vi "CRYReplace Curve Name of Steps.vi"(7 "Option flg":bool, 8 "Steps In":T1[](array[typedef]) {"Repeat State Array"."Start" format="%#_5g"; "Y dB ref" format="%.1f"; "Y data" items=["dB", "Lin"]; "Start" format="%#_5g"}, 9 "Step Category":string, 10 "New Name":string[](array[string]), 11 "Old Name":string[](array[string])) -> (3 "Steps Out":T1[](array[typedef]) {"Repeat State Array"."Start" format="%#_5g"; "Y dB ref" format="%.1f"; "Y data" items=["dB", "Lin"]; "Start" format="%#_5g"})   [LabVIEW 2013]
uses:
  Typedef Control/CRYStep.ctl
  CRYProject/CRYProject Editor Global.vi
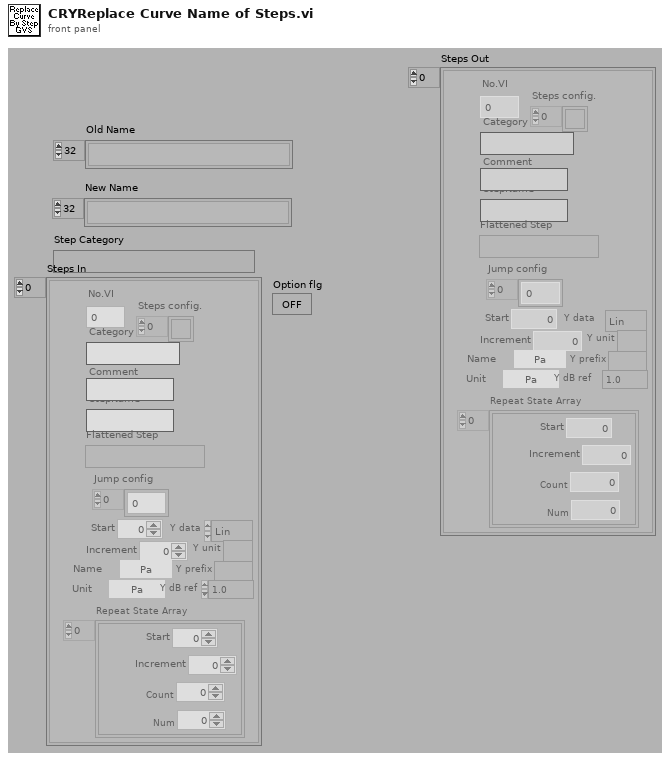
[diagram p1: front panel]
types:
  T1 = typedef "CRYStep.ctl" = cluster{"No.VI":i32, "Category":string, "StepName":string, "Seq setup flattened":string, "Comment":string, "Steps config.":bool[], "Jump config":i32[], "Start":dbl, "Increment":dbl, "Name":string, "Unit":string, "Y data":u16, "Y prefix":string, "Y dB ref":dbl, "Y unit":string, "Repeat State Array":cluster{"Start":dbl, "Increment":dbl, "Count":i32, "Num":i32}[]}
  T2 = typedef "CRYAcquisition Cluster.ctl" = cluster{"Mode":u16, "Name":string, "use ch name":bool, "Record Time":dbl, "hide rec":bool, "hide play":bool, "rec delay":dbl, "rec pad":dbl, "dcc units":i8, "sine gen setting":string, "scope_fft setting":string, "voltmeter setting":string, "rta setting":string, "trig offset(sec)":dbl, "triggered  record":bool, "trig level":dbl, "trig unit":u8, "trig slop":bool, "trig timeout(sec)":dbl, "add record":bool, "EQ":bool, "record table":string[][], "play table":string[][], "trig channel":string, "Help":string}
  T3 = typedef "CRYAnalysis Cluster.ctl" = cluster{"Name":string, "Harmonics":dbl[], " Algorithm":u16, "delay":dbl, "THD(%)":bool, "Rub&Buzz":bool, "Imp":bool, "Imp Ref resistor":dbl, "Y data":u16, "Y prefix":string, "Y unit":string, "Y dB ref":dbl, "Custom Curve Names":string[], "har list items":string[], "Envelope":bool, "use custom unit":bool, "autodelay ch":dbl, "impulse":bool, " start ms":dbl, " stop ms":dbl, "Scaling":i32, "Default Overlap ":bool, "Advanced View":bool, "Loose Particle":bool, "Use default":bool, "Auto-Correlation(Stimulus)":bool, "Auto-Correlation(Response)":bool, "Deconvolved Response":bool, "Mic Current":bool, "M List Vaiues":u16, "Type":u16, "Delay Method":u16, "Apply Correction Out":bool, "Apply Correction In":bool, "Harmonics @ meas.frq":bool, "THD Normalized(%)":bool, "Total Distortion":bool, "THD+Noise(%)":bool, "Rub&Buzz Norm'd(%)":bool, "Standard Error":bool, "Confidence Limits":bool, "Total Diff":bool, "Total Noise":bool, "Total DFD(%)":bool, "Total IMD(%)":bool, "Total IM":bool, "Total DFD+Noise(%)":bool, "Use Channel Name":bool, "Waveform In":string, "Waveform Out":string, "Method":u16, "Spectral Scaling":u16, "Appliied Unit":u16, "Length Unit":u16, "Applied Units":u16, "Sens Item":u16, "Tab":i32, "Distance Unit":u16, "discard cycles":dbl, "Weigting":string, "Averaging Time":dbl, "Max duration":dbl, "Min duration":dbl, "Attack Threshold":dbl, "Hysteresis Up":dbl, "Fmin(Hz)":dbl, "Fmax(Hz)":dbl, "Freq.Resolution":dbl, "Over-samples Res.":dbl, "Win Resolution":dbl, "distance":dbl, "samples":dbl, "Overlap":dbl, "Record Length":dbl, "No.of FFTs":dbl, "Hz":dbl, "record delay":dbl, " Std Err":dbl, "Response":bool, "Coherent Power*":bool, "Stimulus":bool, "Measurement Confidence":bool, "Auto Spectrum(Response)*":bool, "Auto Spectrum(Stimulus)*":bool, "Cross Spectrum*":bool, "functions":bool, "Frequency Response":bool, "Non-Coherent Power*":bool, "Coherence (%)":bool, "Non-Coherence (%)":bool, "Signal-Noise Ratio (dB)":bool, "Non-Coherenct Distirtion*":bool, "Result Waveforms":bool, "Coupling":bool, "Averaging":u16, "Harmonics":i32, "Custom Curve Names":i32, "unLabel":string, "Custom Curve Names":string, "Unit":string, "Total IMD + Noise(%) ":bool, "ResponseMe":u16, "Intermod":dbl[], "Diff\n":dbl[], "Cross-Correlation":bool, "IM list items":string[], "Diff list items":string[], "TSR Window Type":string, "Help":string, "Custom Curve IDs":i32[], "Default Curve Names":string[], "Loose Particle waveform":bool, "Perceptual Rub&Buzz":bool, "Imp Auto Mode":u16, "Mic Auto Mode":u16, "Mic Ref resistor":dbl, "Curve Resolution":u16, "Curve Resolution Hz":dbl, "Polarity":bool}
  T4 = typedef "CRYStimulus Cluster.ctl" = cluster{"StimulusType":string, "UseMLValArray":u16[], "ML_axisArray":u16[], "MLValLevelNameArray":string[], "Level(U)Array":dbl[], "Start(Stop)FreqArray":dbl[], "Start(Stop)AmpArray":dbl[], "StepResolutionArray":u16[], "Unit_Array":u16[], "DegValArray":dbl[], "DegUnitArray":string[], "Steps1":i32, "Cycle/step1(#)":u32, "Time/step1(s)":dbl, "Transition1":dbl, "SweepRate2":dbl, "Freq3(Hz)":dbl, "Steps3(#)":dbl, "Cycles3(#)":u32, "StepSize3":dbl, "wave time":string, "RMS_Value4":dbl, "Peak_Value4":dbl, "WavePath4":string, "RMS_unit4":string, "Peak_unit4":string, "wave Info":string, "dc_ctrl5_1":u16, "dc_ctrl5_2":u16, "dc_polar5":u16, "Max.Current":u16, "Steps5(#)":u32, "Time/Step5":dbl, "Level5":dbl, "StepsSize5Val":dbl, "StepSize5Unit":string, "SweepType":u16, "Fixed/Ratio6":u16, "Transition6":dbl, "Steps6(#)":dbl, "Cycle/Steps6(#)":u32, "Time/Steps6(s)":dbl, "Freq6(Hz)":dbl, "Difference6(Hz)":dbl, "Ratio6":string, "NoiseType7":u16, "Duration7(s)":dbl, "MinFreq7(Hz)":dbl, "MaxFreq7(Hz)":dbl, "MinFreq8(Hz)":dbl, "MaxFreq8(Hz)":dbl, "FreqRounding8":bool, "Duration8(s)":dbl, "Tones8":dbl, "RoundingVal8":dbl, "ApplyEQ":bool, "Duration(s)":dbl, "CustomStimulusName ":string, "Flatten Element Array":string[], "sine waves":cluster{"freq":dbl, "ampl":dbl, "cycles":dbl}[], "Channel Out":i32, "RatioVal6":dbl, "TabCtrl6":enum32{"Master Tone", "Slave Tone"}, "Signal Type Name":string, "Help":string, "Channel Sel":u16, "V on DUT":bool, "Output Imp":dbl, "Nominal Imp":dbl}
  T5 = typedef "CRYLimits.ctl" = cluster{"Name":string, "Tolerance":u16, "X Axis":u16, "Limits":u16, "Upper Limit":cluster{dbl, dbl}[], "Align Ref":cluster{dbl, dbl}, "Lower Limit":cluster{dbl, dbl}[], "Y data":u16, "Y unit":string, "Y dB ref":dbl, "Curve Names":string[], "Y-Resolution":u8, "Type":u16, "x float":bool, "X min-max-step":cluster{"Limit X Offset Min":dbl, "Limit X Offset Max":dbl, "Limit X Offset Step Size":dbl}, "magn/phase":u16, "Upper Limit Type":u16, "Lower Limit Type":u16, "Lim Curve axis up":u16, "Lim Curve axis lo":u16, "Data Selection Upper":u16, "Data Selection Lower":u16, "X-Resolution":u8, "Output failed point curves?":bool, "X data":u16, "X unit":string, "X dB ref":dbl, "X-Y Graph Set-up":string, "Tab Value":enum32{"Data", "Parameters"}, "Help":string, "X Up Val":dbl, "Y Up Val":dbl, "X Low Val":dbl, "Y Low Val":dbl, "Up Limit Val":dbl, "Low Limit Val":dbl, "bAdd DataName":bool, "Custom Name":string}
  T6 = typedef "CRYStatistic cluster.ctl" = cluster{"Mode":u16, "No.Ranked(BF)":i32, "No.Ranked(WF)":i32, "Absolute Margin Standard Deviation":bool, "+/- sigma Res":i32, "Margin Standard Deviation":bool, "Margin Mean":bool, "Overall Yield":bool, "Individual Limits Yield":bool, "LSL Unit":string, "USL Unit\n":string, "LSL":dbl, "USL":dbl, "Worst Fit to Average":bool, "Best Fit to Average":bool, "Ppk":bool, "Pp":bool, "Absolute Standard Deviation":bool, "+/- sigma Dat":i32, "Standard Deviation ":bool, "Mean":bool, "Min ":bool, "Max ":bool, "No.of Curves Selected":i32, "Curves":string[], " Results":string[], "Name":string, "Help":string, "Tab Value":enum32{"Setting", "Help"}, "Work in":u16, "Mode xyz":u16}
  T7 = typedef "CRYPost Processing Cluster.ctl" = cluster{"Name":string, "Op Type":u16, "Curve A":string, "Curve B":string, "Axis Mode":u16, "Work Mode":u16, "Width":u16, "Weighting win":u16, "Search Mode":u16, "Freq Mode":u16, "New Sampling Rate":dbl, "Use Default Name":bool, "x":bool, "y":bool, "z":bool, "All points":bool, "A_single val axis":u16, "B_single val axis":u16, "Use Default Value":bool, "Result Name":string, "Smoothing Width":i32, "Window":u16, "Para_dB":sgl, "Para_%":sgl, "Exponent":sgl, "Hz":dbl, "Direct Weighting":bool, "Auto Inc":bool, "Inc(deg)":i32, "Total Rotation":i32, "Ref Freq Mode":u16, "Ref Waveform":string, "Sampling Rate":dbl, "Weighting Curve":string, "Ref Freq":dbl, "Curve Group":string[], "Search Items":string[], "Custom unit info":cluster{"use custom":bool, "lin/log":u16, "unit":string, "dB ref":dbl, "common dB":u16}, "Unit":string, "Type A":enum16{"Curves", "Values", "Results", "WFM"}, "Type B":enum16{"Curves", "Values", "Results", "WFM"}, "Unary Operator":u16, "Binary Operator":u16, "Statistical Operator":u16, "Constant ":dbl, "New Resolution":u16, "user equation cluster":T8, "Help":string, "Tab Value":enum32{"Setting", "Help"}, "Zwciker_X-axis":u16, "Zwicker_spectrum":bool, "Freq Sampling Mode":u16, "Freq Sampling Rate":dbl, "Smoothing":bool, "Work in Statics":u16, "Result Data":string[]}
  T8 = typedef "CRYUser Equation Cluster.ctl" = cluster{"Custom unit input array":cluster{"use custom":bool, "lin/log":u16, "unit":string, "dB ref":dbl, "common dB":u16}[], "Custom unit results array ":cluster{"use custom":bool, "lin/log":u16, "unit":string, "dB ref":dbl, "common dB":u16}[], "Desired Result Variables":string[], "Desired Result Names":string[], "Input Curve Names":string[], "Input Curve Variables":string[], "equation":string, "Input axis":u16[], "Results axis":u16[], "# input curves":i32, "# Desired result curves ":i32, "Input Values":string[], "Result Values":string[]}
  T9 = typedef "CRYTS.ctl" = cluster{"No.TS":u16, "TS File Path":path, "TS Name":string, "EditStepName":string, "Steps":T1[], "New State":bool, "Change State":bool, "Flattened CurveLib Data":string, "Document Data":string, "EditStepNo":u16, "Operator Start File":string, "Sequence Type":string, "Sequence Language":string}
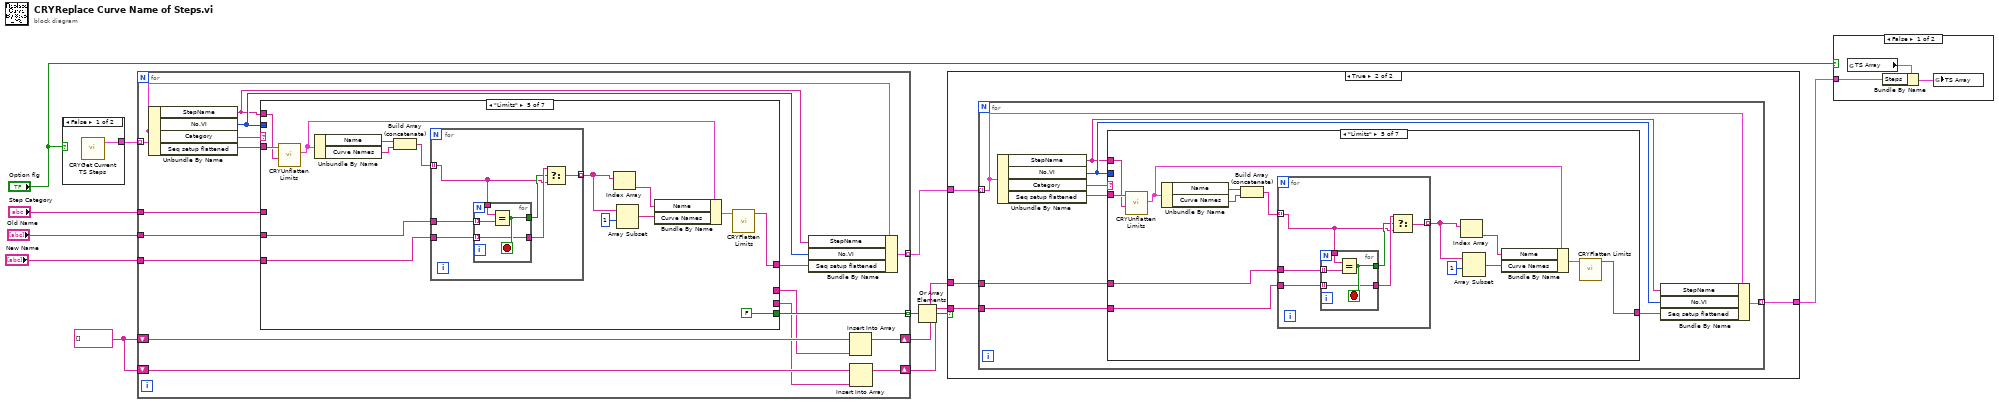
[diagram p0: block diagram]
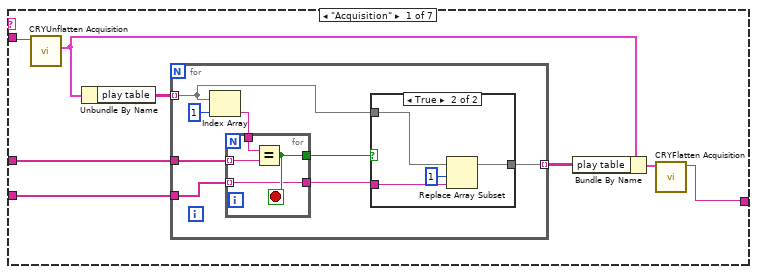
[diagram p3: hidden frame]
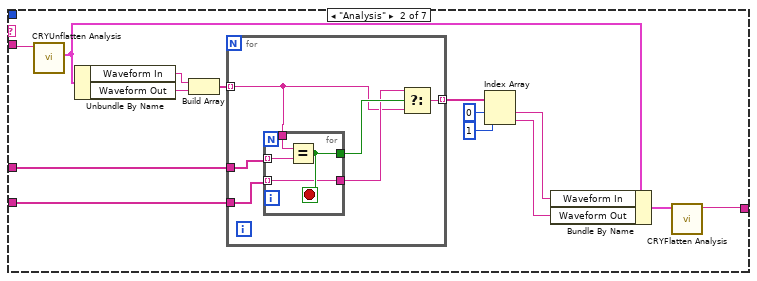
[diagram p5: hidden frame]
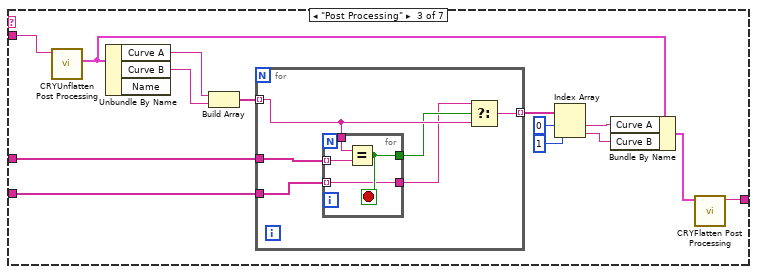
[diagram p6: hidden frame]
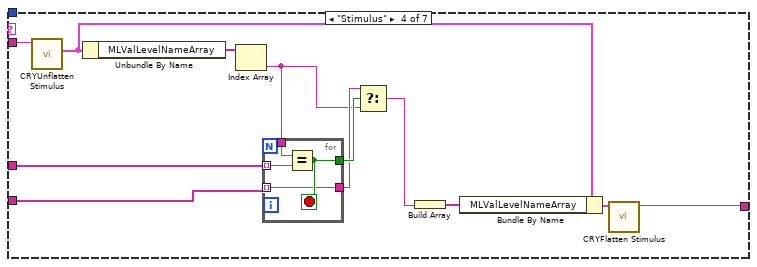
[diagram p7: hidden frame]
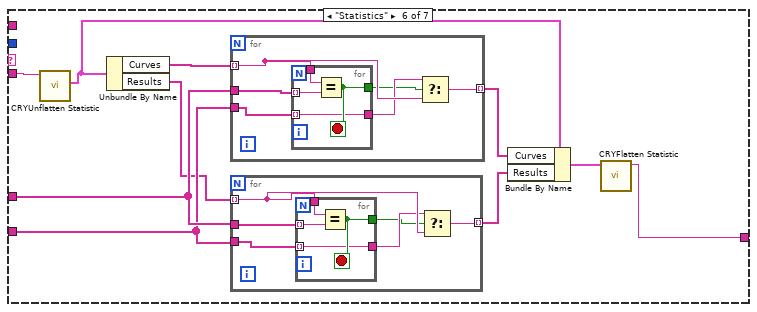
[diagram p8: hidden frame]
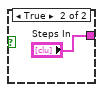
[diagram p10: hidden frame]
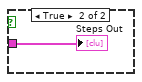
[diagram p11: hidden frame]
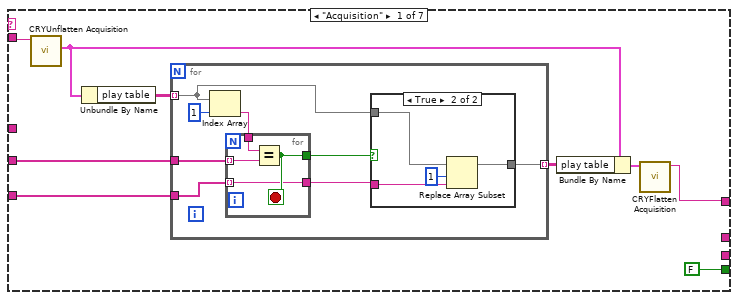
[diagram p12: hidden frame]
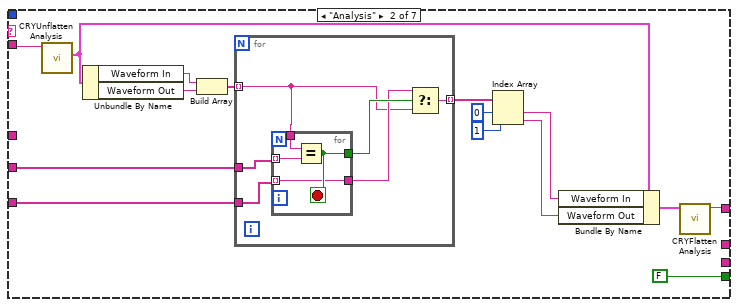
[diagram p14: hidden frame]
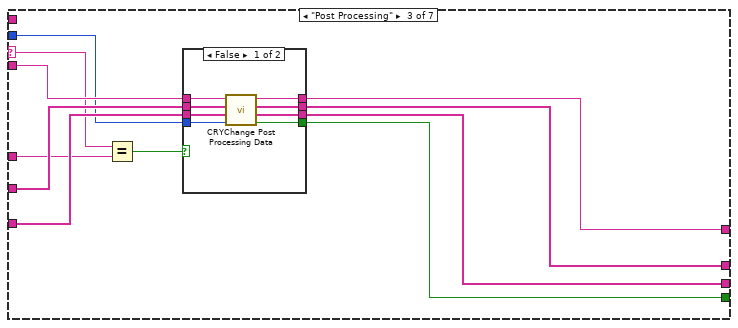
[diagram p15: hidden frame]
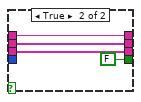
[diagram p16: hidden frame]
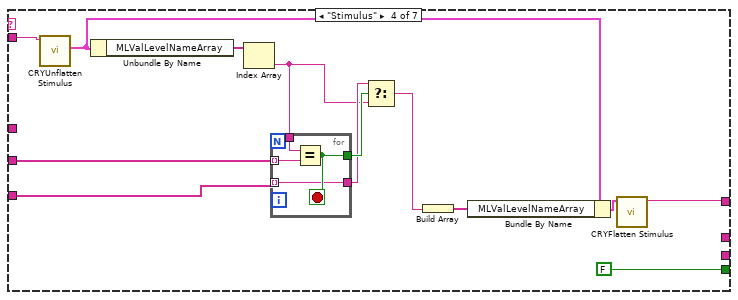
[diagram p17: hidden frame]
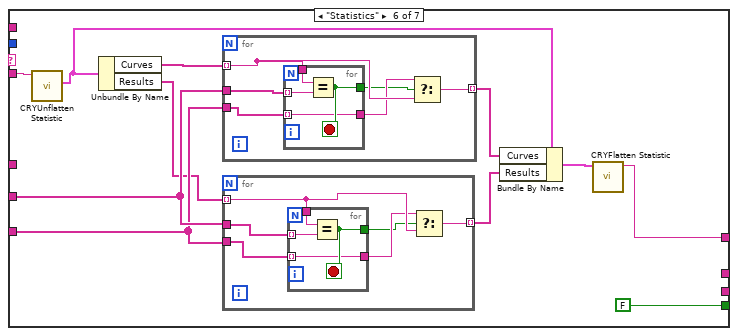
[diagram p18: hidden frame]
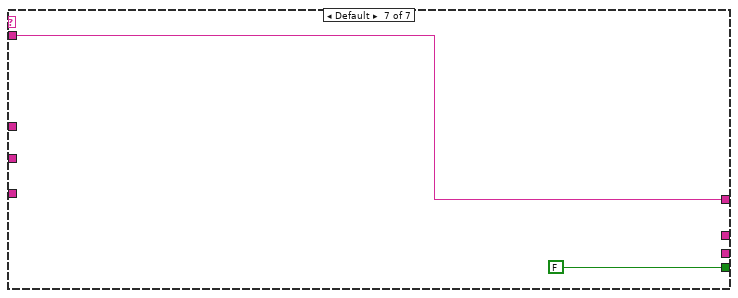
[diagram p19: hidden frame]
diagram:
  w8 = string[] [] ("Inserted Names Out")
  n1 = case shown="False" "Option flg" {
    tunnel: [w13 "Steps In"] -> w10
    frame False {
      n2 = call "CRYGet Current TS Steps.vi"() -> ("Steps"=w13:T1[])  [unwired: 7 in, 4 out]
    }
    frame True {
    }
  }
  n3 = for {
    tunnel: w10 -> [w27] mode=indexing
    tunnel: "Old Name" -> [w29]
    tunnel: "New Name" -> [w28]
    tunnel: [w25] -> w7 mode=indexing
    tunnel: [w23] -> w3 mode=indexing
    shift-right: [w21] -> w6
    shift-left: w8 -> [w22]
    shift-right: [w18] -> w5
    shift-left: w8 -> [w19]
    tunnel: "Step Category" -> [w16]
    n4 = Unbundle By Name(w27) -> ("StepName"=w15:string, "No.VI"=w24:i32, "Category"=w31:string, "Seq setup flattened"=w30:string)
    n5 = case shown="\"Limits\"" w31 {
      selector: w31 -> [_ _ w85 _ _ _ _]
      tunnel: w30 -> [w38 w72 w93 w115 w137 w158 w180]
      tunnel: w29 -> [w40 w70 w92 w118 w136 w156 _]
      tunnel: w28 -> [w39 w69 w91 w117 w135 w155 _]
      tunnel: [w37 w71 w89 w116 w134 w157 w180] -> w26
      tunnel: w24 -> [_ _ w90 _ _ _ _]
      tunnel: [FALSE ("Use Default Value") FALSE ("Use Default Value") w87 FALSE ("Use Default Value") FALSE ("Use Default Value") FALSE ("Use Default Value") FALSE ("Use Default Value")] -> w23
      tunnel: [_ _ w88 _ _ _ _] -> w20
      tunnel: [_ _ w86 _ _ _ _] -> w17
      tunnel: w16 -> [_ _ w84 _ _ _ _]
      tunnel: w15 -> [_ _ _ _ w123 _ _]
      frame "Acquisition" {
        n6 = call "CRYUnflatten Acquisition.vi"("Flatten Acquisition"=w38) -> ("Acquisition"=w36:T2)  [unwired: 8 in, 2 out]
        n7 = Unbundle By Name(w36) -> ("play table"=w34:string[][])
        n8 = for {
          tunnel: w34 -> [w45] mode=indexing
          tunnel: w40 -> [w48]
          tunnel: w39 -> [w42]
          tunnel: [w44] -> w33 mode=indexing
          n9 = Index Array(array=w45, index=1) -> (element=w46:string)
          n10 = for {
            tunnel: w48 -> [w52] mode=indexing
            tunnel: [w50] -> w47
            tunnel: w46 -> [w51]
            tunnel: [w49] -> w41
            tunnel: w42 -> [w49] mode=indexing
            stop <- w50 stop-if-true
            n11 = Equal?(x=w51, y=w52) -> (x = y?=w50:bool)
          }
          n12 = case shown="True" w47 {
            tunnel: w45 -> [w53 w57]
            tunnel: w41 -> [_ w56]
            tunnel: [w53 w55] -> w44
            frame False {
            }
            frame True {
              n13 = Replace Array Subset(array=w57, new element=w56, index=1) -> (w55:string[])
            }
          }
        }
        n14 = Bundle By Name(cluster=w36, "play table"=w33) -> (w35:T2)
        n15 = call "CRYFlatten Acquisition.vi"("Acquisition"=w35) -> ("Acquisition flattened"=w37:string)  [unwired: 10 in]
      }
      frame "Analysis" {
        n16 = call "CRYUnflatten Analysis.vi"("Unflatten Analysis"=w72) -> ("Analysis"=w68:T3)  [unwired: 8 in, 2 out]
        n17 = Unbundle By Name(w68) -> ("Waveform In"=w66:string, "Waveform Out"=w65:string)
        n18 = Build Array(w66, w65) -> (w64:string[])
        n19 = for {
          tunnel: w64 -> [w73] mode=indexing
          tunnel: w70 -> [w77]
          tunnel: [w78] -> w63 mode=indexing
          tunnel: w69 -> [w76]
          n20 = for {
            tunnel: w77 -> [w82] mode=indexing
            tunnel: [w80] -> w75
            tunnel: w73 -> [w81]
            tunnel: [w79] -> w74
            tunnel: w76 -> [w79] mode=indexing
            stop <- w80 stop-if-true
            n21 = Equal?(x=w81, y=w82) -> (x = y?=w80:bool)
          }
          n22 = Select(t=w74, s=w75, f=w73) -> (s? t:f=w78:string)
        }
        n23 = Index Array(array=w63, index #1=0 ("index"), index #2=1 ("index")) -> (element #1=w60:string, element #2=w59:string)
        n24 = Bundle By Name(cluster=w68, "Waveform In"=w60, "Waveform Out"=w59) -> (w67:T3)
        n25 = call "CRYFlatten Analysis.vi"("Analysis"=w67) -> ("Analysis flattened"=w71:string)  [unwired: 10 in]
      }
      frame "Post Processing" {
        n26 = Equal?(x=w85, y=w84) -> (x = y?=w83:bool)
        n27 = case shown="False" w83 {
          tunnel: w93 -> [w101 w105]
          tunnel: w92 -> [w100 w104]
          tunnel: w91 -> [w99 w103]
          tunnel: w90 -> [w98 _]
          tunnel: [w97 w105] -> w89
          tunnel: [w96 w104] -> w88
          tunnel: [w95 FALSE ("Use Default Value")] -> w87
          tunnel: [w94 w103] -> w86
          frame False {
            n28 = call "CRYChange Post Processing Data.vi"("Step Setup VI No"=w98, "New Name"=w99, "Old Name"=w100, "Flatten Post Processing"=w101) -> ("Use Default Value"=w95:bool, "Inserted Names Out"=w94:string[], "Original Names Out"=w96:string[], "Post Processing flattened Out"=w97:string)  [unwired: 4 in]
          }
          frame True {
          }
        }
      }
      frame "Stimulus" {
        n29 = call "CRYUnflatten Stimulus.vi"("Flatten Stimulus"=w115) -> ("Stimulus"=w114:T4)  [unwired: 8 in, 2 out]
        n30 = Unbundle By Name(w114) -> ("MLValLevelNameArray"=w112:string[])
        n31 = Index Array(array=w112) -> (element=w107:string)  [unwired: 1 in]
        n32 = for {
          tunnel: w118 -> [w122] mode=indexing
          tunnel: [w120] -> w109
          tunnel: w107 -> [w121]
          tunnel: [w119] -> w108
          tunnel: w117 -> [w119] mode=indexing
          stop <- w120 stop-if-true
          n33 = Equal?(x=w121, y=w122) -> (x = y?=w120:bool)
        }
        n34 = Select(t=w108, s=w109, f=w107) -> (s? t:f=w111:string)
        n35 = Build Array(w111) -> (w110:string[])
        n36 = Bundle By Name(cluster=w114, "MLValLevelNameArray"=w110) -> (w113:T4)
        n37 = call "CRYFlatten Stimulus.vi"("Stimulus"=w113) -> ("Flatten Stimulus String"=w116:string)  [unwired: 10 in]
      }
      frame "Limits" {
        n38 = call "CRYUnflatten Limits.vi"("Step Name"=w123, "Unflatten Limits"=w137) -> ("Limits"=w125:T5)  [unwired: 7 in, 2 out]
        n39 = Unbundle By Name(w125) -> ("Name"=w133:string, "Curve Names"=w132:string[])
        n40 = Build Array (concatenate)(w133, w132) -> (w131:string[])
        n41 = for {
          tunnel: w131 -> [w138] mode=indexing
          tunnel: w136 -> [w142]
          tunnel: [w143] -> w128 mode=indexing
          tunnel: w135 -> [w141]
          n42 = for {
            tunnel: w142 -> [w147] mode=indexing
            tunnel: [w145] -> w139
            tunnel: w138 -> [w146]
            tunnel: [w144] -> w140
            tunnel: w141 -> [w144] mode=indexing
            stop <- w145 stop-if-true
            n43 = Equal?(x=w146, y=w147) -> (x = y?=w145:bool)
          }
          n44 = Select(t=w140, s=w139, f=w138) -> (s? t:f=w143:string)
        }
        n45 = Index Array(array=w128) -> (element=w129:string)  [unwired: 1 in]
        n46 = Array Subset(array=w128, index=1) -> (w126:string[])  [unwired: 1 in]
        n47 = Bundle By Name(cluster=w125, "Name"=w129, "Curve Names"=w126) -> (w130:T5)
        n48 = call "CRYFlatten Limits.vi"("Limits"=w130) -> ("Flatten Limits String"=w134:string)  [unwired: 10 in]
      }
      frame "Statistics" {
        n49 = call "CRYUnflatten Statistic.vi"("Flatten Statistics"=w158) -> ("Statistics"=w149:T6)  [unwired: 8 in, 2 out]
        n50 = Unbundle By Name(w149) -> ("Curves"=w153:string[], "Results"=w151:string[])
        n51 = for {
          tunnel: w153 -> [w173] mode=indexing
          tunnel: w156 -> [w172]
          tunnel: [w174] -> w152 mode=indexing
          tunnel: w155 -> [w171]
          n52 = for {
            tunnel: w172 -> [w178] mode=indexing
            tunnel: [w176] -> w169
            tunnel: w173 -> [w177]
            tunnel: [w175] -> w170
            tunnel: w171 -> [w175] mode=indexing
            stop <- w176 stop-if-true
            n53 = Equal?(x=w177, y=w178) -> (x = y?=w176:bool)
          }
          n54 = Select(t=w170, s=w169, f=w173) -> (s? t:f=w174:string)
        }
        n55 = for {
          tunnel: w151 -> [w161] mode=indexing
          tunnel: w156 -> [w163]
          tunnel: [w164] -> w150 mode=indexing
          tunnel: w155 -> [w162]
          n56 = for {
            tunnel: w163 -> [w168] mode=indexing
            tunnel: [w166] -> w159
            tunnel: w161 -> [w167]
            tunnel: [w165] -> w160
            tunnel: w162 -> [w165] mode=indexing
            stop <- w166 stop-if-true
            n57 = Equal?(x=w167, y=w168) -> (x = y?=w166:bool)
          }
          n58 = Select(t=w160, s=w159, f=w161) -> (s? t:f=w164:string)
        }
        n59 = Bundle By Name(cluster=w149, "Curves"=w152, "Results"=w150) -> (w154:T6)
        n60 = call "CRYFlatten Statistic.vi"("Statistics"=w154) -> ("Flatten Statistics String"=w157:string)  [unwired: 10 in]
      }
      frame Default {
      }
    }
    n61 = Bundle By Name(cluster=w27, "StepName"=w15, "No.VI"=w24, "Seq setup flattened"=w26) -> (w25:T1)
    n62 = Insert Into Array(array=w22, new element=w20) -> (w21:string[])  [unwired: 1 in]
    n63 = Insert Into Array(array=w19, new element=w17) -> (w18:string[])  [unwired: 1 in]
  }
  n64 = Or Array Elements(Boolean array=w3) -> (logical OR=w2:bool)
  n65 = case shown="True" w2 {
    tunnel: w7 -> [w181 w185]
    tunnel: w6 -> [_ w184]
    tunnel: w5 -> [_ w183]
    tunnel: [w181 w182] -> w4
    frame False {
    }
    frame True {
      n66 = for {
        tunnel: w185 -> [w190] mode=indexing
        tunnel: w184 -> [w192]
        tunnel: w183 -> [w191]
        tunnel: [w188] -> w182 mode=indexing
        n67 = Unbundle By Name(w190) -> ("StepName"=w186:string, "No.VI"=w187:i32, "Category"=w194:string, "Seq setup flattened"=w193:string)
        n68 = case shown="\"Limits\"" w194 {
          tunnel: w193 -> [w200 w233 w251 w276 w297 w317 w338]
          tunnel: w192 -> [w202 w231 w248 w279 w296 w315 _]
          tunnel: w191 -> [w201 w230 w247 w278 w295 w314 _]
          tunnel: [w199 w232 w244 w277 w294 w316 w338] -> w189
          tunnel: w187 -> [_ _ _ _ _ _ _]
          tunnel: w186 -> [_ _ _ _ w284 _ _]
          frame "Acquisition" {
            n69 = call "CRYUnflatten Acquisition.vi"("Flatten Acquisition"=w200) -> ("Acquisition"=w198:T2)  [unwired: 8 in, 2 out]
            n70 = Unbundle By Name(w198) -> ("play table"=w196:string[][])
            n71 = for {
              tunnel: w196 -> [w207] mode=indexing
              tunnel: w202 -> [w210]
              tunnel: w201 -> [w204]
              tunnel: [w206] -> w195 mode=indexing
              n72 = Index Array(array=w207, index=1) -> (element=w208:string)
              n73 = for {
                tunnel: w210 -> [w214] mode=indexing
                tunnel: [w212] -> w209
                tunnel: w208 -> [w213]
                tunnel: [w211] -> w203
                tunnel: w204 -> [w211] mode=indexing
                stop <- w212 stop-if-true
                n74 = Equal?(x=w213, y=w214) -> (x = y?=w212:bool)
              }
              n75 = case shown="True" w209 {
                tunnel: w207 -> [w215 w219]
                tunnel: w203 -> [_ w218]
                tunnel: [w215 w217] -> w206
                frame False {
                }
                frame True {
                  n76 = Replace Array Subset(array=w219, new element=w218, index=1) -> (w217:string[])
                }
              }
            }
            n77 = Bundle By Name(cluster=w198, "play table"=w195) -> (w197:T2)
            n78 = call "CRYFlatten Acquisition.vi"("Acquisition"=w197) -> ("Acquisition flattened"=w199:string)  [unwired: 10 in]
          }
          frame "Analysis" {
            n79 = call "CRYUnflatten Analysis.vi"("Unflatten Analysis"=w233) -> ("Analysis"=w229:T3)  [unwired: 8 in, 2 out]
            n80 = Unbundle By Name(w229) -> ("Waveform In"=w227:string, "Waveform Out"=w226:string)
            n81 = Build Array(w227, w226) -> (w225:string[])
            n82 = for {
              tunnel: w225 -> [w234] mode=indexing
              tunnel: w231 -> [w238]
              tunnel: [w239] -> w224 mode=indexing
              tunnel: w230 -> [w237]
              n83 = for {
                tunnel: w238 -> [w243] mode=indexing
                tunnel: [w241] -> w236
                tunnel: w234 -> [w242]
                tunnel: [w240] -> w235
                tunnel: w237 -> [w240] mode=indexing
                stop <- w241 stop-if-true
                n84 = Equal?(x=w242, y=w243) -> (x = y?=w241:bool)
              }
              n85 = Select(t=w235, s=w236, f=w234) -> (s? t:f=w239:string)
            }
            n86 = Index Array(array=w224, index #1=0 ("index"), index #2=1 ("index")) -> (element #1=w221:string, element #2=w220:string)
            n87 = Bundle By Name(cluster=w229, "Waveform In"=w221, "Waveform Out"=w220) -> (w228:T3)
            n88 = call "CRYFlatten Analysis.vi"("Analysis"=w228) -> ("Analysis flattened"=w232:string)  [unwired: 10 in]
          }
          frame "Post Processing" {
            n89 = call "CRYUnflatten Post Processing.vi"("Unflatten Post Processing"=w251) -> ("Post-Processing"=w246:T7)  [unwired: 8 in, 2 out]
            n90 = Unbundle By Name(w246) -> ("Curve A"=w250:string, "Curve B"=w249:string)  [unwired: 1 out]
            n91 = Build Array(w250, w249) -> (w257:string[])
            n92 = for {
              tunnel: w257 -> [w260] mode=indexing
              tunnel: w248 -> [w262]
              tunnel: [w263] -> w256 mode=indexing
              tunnel: w247 -> [w261]
              n93 = for {
                tunnel: w262 -> [w267] mode=indexing
                tunnel: [w265] -> w259
                tunnel: w260 -> [w266]
                tunnel: [w264] -> w258
                tunnel: w261 -> [w264] mode=indexing
                stop <- w265 stop-if-true
                n94 = Equal?(x=w266, y=w267) -> (x = y?=w265:bool)
              }
              n95 = Select(t=w258, s=w259, f=w260) -> (s? t:f=w263:string)
            }
            n96 = Index Array(array=w256, index #1=0 ("index"), index #2=1 ("index")) -> (element #1=w253:string, element #2=w252:string)
            n97 = Bundle By Name(cluster=w246, "Curve A"=w253, "Curve B"=w252) -> (w245:T7)
            n98 = call "CRYFlatten Post Processing.vi"("Post-Processing"=w245) -> ("Post Processing flattened"=w244:string)  [unwired: 10 in]
          }
          frame "Stimulus" {
            n99 = call "CRYUnflatten Stimulus.vi"("Flatten Stimulus"=w276) -> ("Stimulus"=w275:T4)  [unwired: 8 in, 2 out]
            n100 = Unbundle By Name(w275) -> ("MLValLevelNameArray"=w273:string[])
            n101 = Index Array(array=w273) -> (element=w268:string)  [unwired: 1 in]
            n102 = for {
              tunnel: w279 -> [w283] mode=indexing
              tunnel: [w281] -> w270
              tunnel: w268 -> [w282]
              tunnel: [w280] -> w269
              tunnel: w278 -> [w280] mode=indexing
              stop <- w281 stop-if-true
              n103 = Equal?(x=w282, y=w283) -> (x = y?=w281:bool)
            }
            n104 = Select(t=w269, s=w270, f=w268) -> (s? t:f=w272:string)
            n105 = Build Array(w272) -> (w271:string[])
            n106 = Bundle By Name(cluster=w275, "MLValLevelNameArray"=w271) -> (w274:T4)
            n107 = call "CRYFlatten Stimulus.vi"("Stimulus"=w274) -> ("Flatten Stimulus String"=w277:string)  [unwired: 10 in]
          }
          frame "Limits" {
            n108 = call "CRYUnflatten Limits.vi"("Step Name"=w284, "Unflatten Limits"=w297) -> ("Limits"=w285:T5)  [unwired: 7 in, 2 out]
            n109 = Unbundle By Name(w285) -> ("Name"=w293:string, "Curve Names"=w292:string[])
            n110 = Build Array (concatenate)(w293, w292) -> (w291:string[])
            n111 = for {
              tunnel: w291 -> [w298] mode=indexing
              tunnel: w296 -> [w302]
              tunnel: [w303] -> w288 mode=indexing
              tunnel: w295 -> [w301]
              n112 = for {
                tunnel: w302 -> [w307] mode=indexing
                tunnel: [w305] -> w299
                tunnel: w298 -> [w306]
                tunnel: [w304] -> w300
                tunnel: w301 -> [w304] mode=indexing
                stop <- w305 stop-if-true
                n113 = Equal?(x=w306, y=w307) -> (x = y?=w305:bool)
              }
              n114 = Select(t=w300, s=w299, f=w298) -> (s? t:f=w303:string)
            }
            n115 = Index Array(array=w288) -> (element=w289:string)  [unwired: 1 in]
            n116 = Array Subset(array=w288, index=1) -> (w286:string[])  [unwired: 1 in]
            n117 = Bundle By Name(cluster=w285, "Name"=w289, "Curve Names"=w286) -> (w290:T5)
            n118 = call "CRYFlatten Limits.vi"("Limits"=w290) -> ("Flatten Limits String"=w294:string)  [unwired: 10 in]
          }
          frame "Statistics" {
            n119 = call "CRYUnflatten Statistic.vi"("Flatten Statistics"=w317) -> ("Statistics"=w308:T6)  [unwired: 8 in, 2 out]
            n120 = Unbundle By Name(w308) -> ("Curves"=w312:string[], "Results"=w310:string[])
            n121 = for {
              tunnel: w312 -> [w332] mode=indexing
              tunnel: w315 -> [w331]
              tunnel: [w333] -> w311 mode=indexing
              tunnel: w314 -> [w330]
              n122 = for {
                tunnel: w331 -> [w337] mode=indexing
                tunnel: [w335] -> w328
                tunnel: w332 -> [w336]
                tunnel: [w334] -> w329
                tunnel: w330 -> [w334] mode=indexing
                stop <- w335 stop-if-true
                n123 = Equal?(x=w336, y=w337) -> (x = y?=w335:bool)
              }
              n124 = Select(t=w329, s=w328, f=w332) -> (s? t:f=w333:string)
            }
            n125 = for {
              tunnel: w310 -> [w320] mode=indexing
              tunnel: w315 -> [w322]
              tunnel: [w323] -> w309 mode=indexing
              tunnel: w314 -> [w321]
              n126 = for {
                tunnel: w322 -> [w327] mode=indexing
                tunnel: [w325] -> w318
                tunnel: w320 -> [w326]
                tunnel: [w324] -> w319
                tunnel: w321 -> [w324] mode=indexing
                stop <- w325 stop-if-true
                n127 = Equal?(x=w326, y=w327) -> (x = y?=w325:bool)
              }
              n128 = Select(t=w319, s=w318, f=w320) -> (s? t:f=w323:string)
            }
            n129 = Bundle By Name(cluster=w308, "Curves"=w311, "Results"=w309) -> (w313:T6)
            n130 = call "CRYFlatten Statistic.vi"("Statistics"=w313) -> ("Flatten Statistics String"=w316:string)  [unwired: 10 in]
          }
          frame Default {
          }
        }
        n131 = Bundle By Name(cluster=w190, "StepName"=w186, "No.VI"=w187, "Seq setup flattened"=w189) -> (w188:T1)
      }
    }
  }
  n132 = case shown="False" "Option flg" {
    tunnel: w4 -> [w339 w342]
    frame False {
      n133 = global read "CRYProject Editor Global.vi" "TS Array"() -> (w341:T9)
      n134 = Bundle By Name(cluster=w341, "Steps"=w339) -> (w340:T9)
      n135 = global write "CRYProject Editor Global.vi" "TS Array"(w340) -> ()
    }
    frame True {
      "Steps Out" <- w342
    }
  }
